vi "Play1.vi"() -> ()   [LabVIEW 2019]
uses:
  HeirDAL Library/Common Library/Controls/Datatype.ctl
  HeirDAL Library/Database Library/Database Manager Class/Controls/Mode.ctl
  HeirDAL Library/Database Library/Sqlite Database Manager/Sqlite Database Manager.lvclass
  G:/DevelopmentEnvironment/LabVIEW Projects/HeirDAL-LV/src/HeirDAL Library/Database Library/Database Manager Class/Database Manager.lvclass
  HeirDAL Library/Models Library/Object Class/Object.lvclass/Object.ctl
  HeirDAL Library/Models Library/Object Class/VIs/Get Name.vi
  HeirDAL Library/Models Library/Object Class/VIs/Get Datatype.vi
  HeirDAL Library/Database Library/Database Manager Class/Database Manager.lvclass
  HeirDAL Library/Database Library/Repositories Library/Objects Class/Objects.lvclass
  HeirDAL Library/Common Library/Common.lvlib
  HeirDAL Library/Models Library/Object Class/Object.lvclass
panel:
  out "Datatype":T1
  out "Name":string
  out "Data Source":string
  out "Rows":map{string, variant}[](array[numeric])
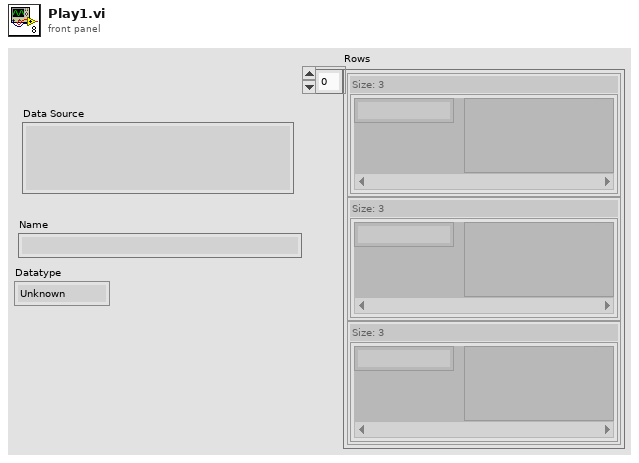
[diagram p1: front panel]
types:
  T1 = typedef "HierDAL Library.lvlib/Common.lvlib/Datatype.ctl" = enum16{"Unknown", "Group", "Dataset"}
  T2 = typedef "HierDAL Library.lvlib/Database.lvlib/Database Manager.lvclass/Mode.ctl" = enum16{"Create", "Replace", "Open", "Read Only"}
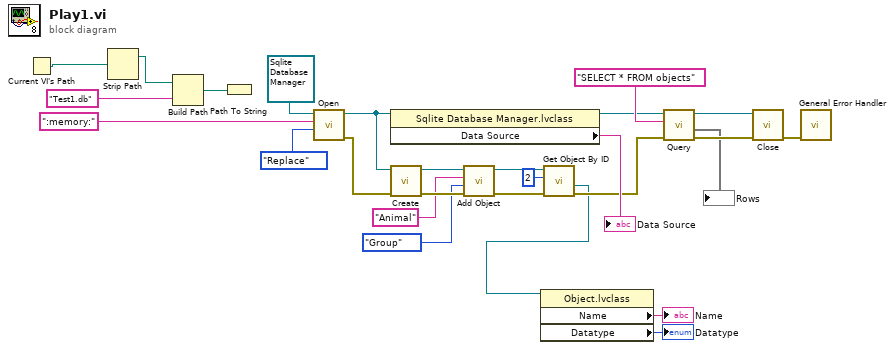
[diagram p0: block diagram]
diagram:
  n1 = Current VI's Path() -> (path=w25:path)
  n2 = Strip Path(path=w25) -> (stripped path=w24:path)  [unwired: 1 out]
  n3 = Build Path(base path=w24, name or relative path="Test1.db") -> (appended path=w26:path)
  n4 = Path To String(path=w26) -> ()  [unwired: 1 out]
  n5 = call-dynamic "Open.vi"("Mode"=Mode."Replace", "Data Source"=":memory:", "Sqlite Database Manager in"=refnum<class "Sqlite Database Manager.lvclass"> refnum) -> ("error out"=w15:errorcluster, "Sqlite Database Manager out"=w10:refnum<class "Sqlite Database Manager.lvclass">)  [unwired: 7 in]
  n6 = property class="Sqlite Database Manager.lvclass"(reference=w10) -> (reference out=w9:refnum<class "Sqlite Database Manager.lvclass">, "Data Source"=→"Data Source":string)  [unwired: 1 in, 1 out]
  n7 = call "Create.vi"("error in (no error)"=w15, "Database Manager"=w10) -> ("error out"=w14:errorcluster, "Objects out"=w13:refnum<class "Objects.lvclass">)  [unwired: 8 in]
  n8 = call "Add Object.vi"("error in (no error)"=w14, "Datatype"=Datatype."Group", "Name"="Animal", "Objects in"=w13) -> ("error out"=w7:errorcluster, "Objects out"=w6:refnum<class "Objects.lvclass">)  [unwired: 6 in]
  n9 = call "Get Object By ID.vi"("error in (no error)"=w7, "ID"=2, "Objects in"=w6) -> ("error out"=w5:errorcluster, "Object"=w3:refnum<class "Object.lvclass">)  [unwired: 6 in, 1 out]
  n10 = property class="Object.lvclass"(reference=w3) -> ("Name"=→"Name":string, "Datatype"=→"Datatype":T1)  [unwired: 1 in, 2 out]
  n11 = call-dynamic "Query.vi"("error in (no error)"=w5, "Query"="SELECT * FROM objects", "Sqlite Database Manager in"=w9) -> ("error out"=w19:errorcluster, "Rows"=→"Rows":map{string, variant}[], "Sqlite Database Manager out"=w18:refnum<class "Sqlite Database Manager.lvclass">)  [unwired: 6 in]
  n12 = call-dynamic "Close.vi"("error in (no error)"=w19, "Sqlite Database Manager in"=w18) -> ("error out"=w21:errorcluster)  [unwired: 9 in]
  n13 = call <vilib>:"General Error Handler.vi"("error in (no error)"=w21) -> ()  [unwired: 10 in, 5 out]
